vi "Duplicate Library.vi"(11 "Path":path) -> (3 "New Library Path":path)   [LabVIEW 2020]
uses:
  <vilib>/regexp/Match Regular Expression.xnode
panel:
  in  "Numer of Copies":i32=7
  # "Use path to library or class with the highest number in the name."
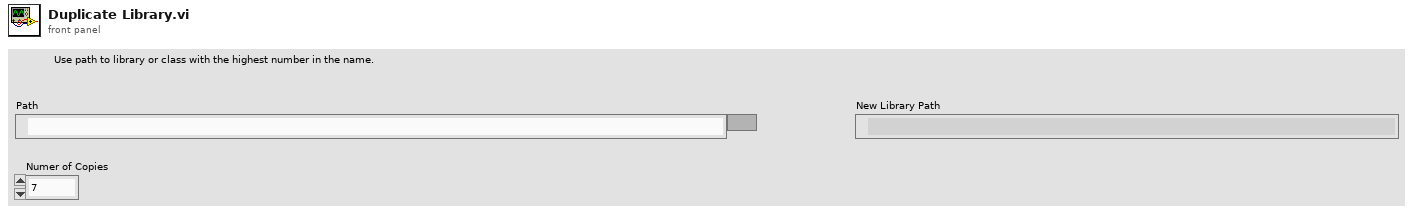
[diagram p1: front panel]
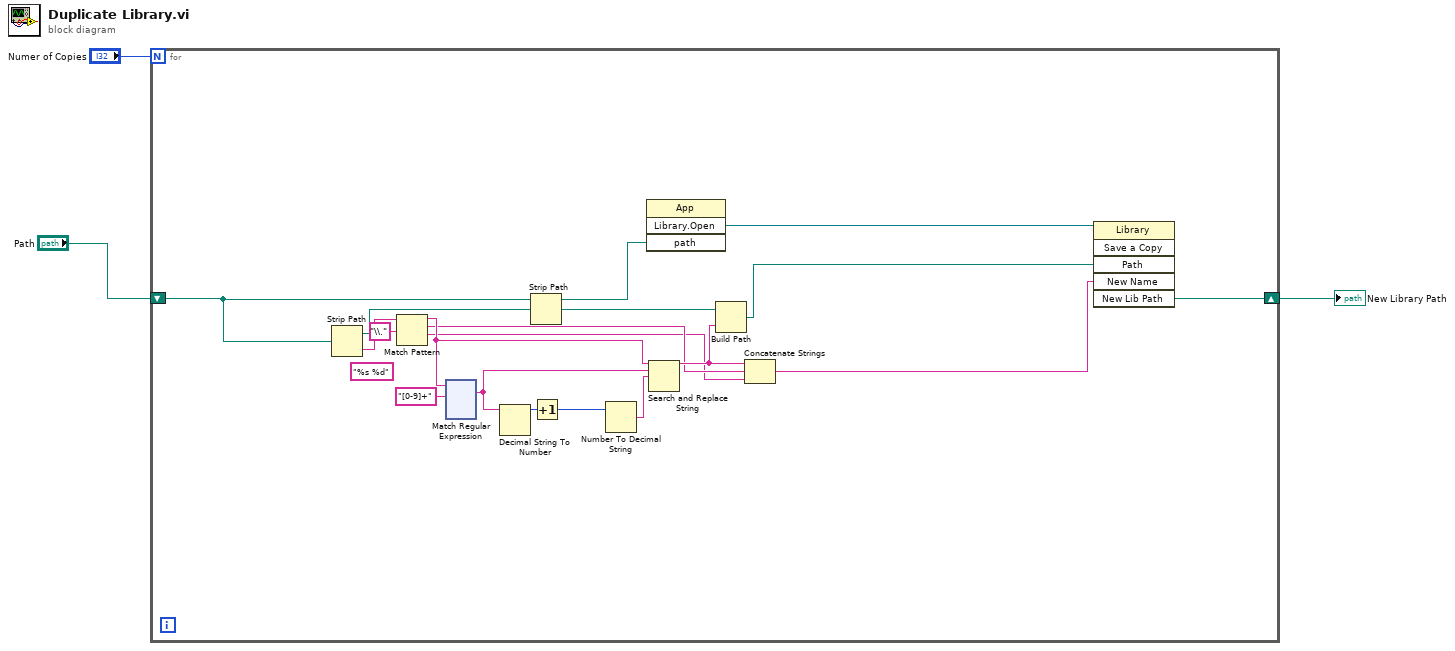
[diagram p0: block diagram]
diagram:
  n1 = for {
    N: "Numer of Copies" -> [_]
    shift-right: [w4] -> w2
    shift-left: "Path" -> [w21]
    (unwired) "%s %d" ("format string")
    n2 = Strip Path(path=w21) -> (stripped path=w19:path, name=w18:string)
    n3 = Match Pattern(string=w18, regular expression="\\.") -> (before substring=w11:string, match substring=w10:string, after substring=w9:string)  [unwired: 1 in, 1 out]
    n4 = xnode "Match Regular Expression"("input string"=w11, "regular expression"="[0-9]+") -> ("whole match"=w15:string)  [unwired: 4 in, 4 out]
    n5 = Decimal String To Number(string=w15) -> (number=w14:i32)  [unwired: 2 in, 1 out]
    n6 = Strip Path(path=w19) -> (stripped path=w8:path)  [unwired: 1 out]
    n7 = Increment(x=w14) -> (x+1=w16:i32)
    n8 = Number To Decimal String(number=w16) -> (decimal integer string=w20:string)  [unwired: 1 in]
    n9 = invoke class="App" method="Library.Open"("path"=w21) -> ("Open Library"=w7:refnum<vi>)  [unwired: 3 in, 3 out]
    n10 = Search and Replace String(input string=w11, search string=w15, replace string=w20) -> (result string=w12:string)  [unwired: 5 in, 3 out]
    n11 = Build Path(base path=w8, name or relative path=w12) -> (appended path=w6:path)
    n12 = Concatenate Strings(w12, w10, w9) -> (w5:string)
    n13 = invoke class="Library" method="Save a Copy"(reference=w7, "Path"=w6, "New Name"=w5) -> ("New Lib Path"=w4:path)  [unwired: 3 in, 5 out]
  }
  "New Library Path" <- w2
